vi "1608fsdr_v2.vi"() -> ()   [LabVIEW 2009]
uses:
  Das16.llb/FromEng(trigger).VI
  Das16.llb/ToEng(array).vi
  PD_Filepath.vi
  Global 2.vi
  Global 3.vi
  DAQGlobal.vi
panel:
  in  "Tab Control":enum32{"Setup", "Acquisition"}(tab)
  in  "Type":u32(ring)=12
  in  "LowThreshold\n             (Volts)":sgl min=-10 max=10 format="%.2f"
  in  "HighThreshold \n              (Volts)":sgl=3.0 min=-10 max=10 format="%.2f"
  out "SetTrig ErrMsg":string
  in  "Mode":i32(ring) items=["DEFAULTIO", "SINGLEIO", "DMAIO", "BLOCKIO", "BURSTIO"]
  in  "Extclock":bool
  in  "BoardNum":u32=1
  in  "Count":i32=1000
  in  "Rate":i32=5000
  in  "LowChan":i32
  in  "HighChan":i32=4
  out "Actual Rate":i32=1000
  in  "Range":i32(ring)=1 items=["Not Programmable"=0, "+- 20 V"=27, "+- 10 V"=1, "+- 5 V"=2, "+- 4 V"=28, "+- 2.5 V"=3, "+- 2 V"=29, "+- 1.67 V"=4, "+- 1.25 V"=5, "+- 1 V"=6, "+- .625 V"=7, "+- .5 V"=8, "+- .25 V"=30, "+- .2 V"=31, "+- .1 V"=9, "+- .05 V"=10, "+- .01 V"=11, "+- .005 V"=12, "0 - 10 V"=13, "0 - 5 V"=14, "0 - 4 V"=36, "0 - 2.5 V"=15, "0 - 2 V"=16, "0 - 1.67 V"=17, "0 - 1.25 V"=18, "0 - 1 V"=19, "0 - .5 V"=32, "0 - .25 V"=33, "0 - .2 V"=34, "0 - .1 V"=20, "0 - .02 V"=35, "0 - .01 V"=21, "4 - 20 mA"=22, "2 - 10 mA"=23, "1 - 5 mA"=24, ".5 - 2.5 mA"=25, "0 - 20 mA"=26]
  in  "InterChannel Delay":dbl=-1.0 format="%.2f"
  in  "ExtTrigger":bool
  out "Count/Channel":u32=500
  out "Channel Count":u32=2
  in  "stop 2":bool
  in  "time format string (%c)":string
  in  "width (-)":i16
  in  "precision (6)":i16
  out "Complete data output path":path=path "C:/Docs/LabVIEW Data/Acquisition.lvm" caption="File Name Out"
  out "Statistics filename":string
  out "Saving?":bool
  out "Streaming data":sgl[][](graph)
  out "Instantaneous data":sgl[][](graph)=[[-0.009002686, -0.00869751, -0.008392334, -0.007019043, -0.0015258789, -0.00793457, -0.0073242188, 0.00076293945, -0.00579834, -0.007171631, 0.0022888184, 0.0048828125, 0.0010681152, 0.008087158, 0.0064086914, -0.0025939941, 0.0033569336, 0.0051879883, -0.007019043, -0.007019043, -0.004119873, 0.0061035156, 0.00015258789, -0.0022888184, -0.0047302246, -0.0064086914, -0.0047302246, 0.0074768066, 0.0074768066, 0.004119873, 0.009002686, 0.008544922, 0.0018310547, 0.00579834, 0.006866455, -0.0032043457, -0.009155273, -0.0032043457, -0.0059509277, 0.00015258789, 0.0032043457, -0.0018310547, -0.00091552734, -0.007019043, 0.0035095215, 0.0051879883, -0.004272461, -0.00579834, -0.006713867, 0.004272461, -0.0036621094, 0.00579834, 0.00030517578, -0.0030517578, 0.0073242188, 0.0015258789, 0.00030517578, -0.007019043, 0.008087158, 0.004119873, -0.007019043, -0.0038146973, -0.00579834, 0.0048828125, 0.0064086914, 0.0073242188, -0.0076293945, -0.00793457, -0.0021362305, 0.00579834, 0.0048828125, -0.00793457, -0.0051879883, -0.00091552734, 0.007171631, 0.003967285, 0.007171631, -0.0047302246, -0.007019043, 0.005340576, 0.008392334, 0.0022888184, -0.0045776367, -0.0015258789, -0.008239746, -0.0030517578, 0.004272461, -0.00030517578, 0.007171631, 0.0048828125, -0.0019836426, 0.0010681152, 0.00030517578, 0.0076293945, 0.00030517578, -0.0030517578, 0.008392334, 0.009002686, 0.008239746, -0.006866455, 0.0018310547, -0.0064086914, -0.0032043457, 0.0010681152, -0.00793457, -0.00061035156, 0.0012207031, 0.0073242188, -0.0061035156, -0.0018310547, 0.0076293945, 0.0024414062, 0.007019043, -0.0050354004, -0.0059509277, -0.00579834, 0.008850098, 0.0064086914, 0.0, -0.009002686, -0.006713867, 0.007171631, 0.0050354004, 0.00076293945, -0.009307861, -0.0010681152, -0.007171631, -0.0032043457, 0.0048828125, -0.00076293945, 0.0045776367, 0.00793457, 0.0048828125, -0.0033569336, 0.001373291, 0.005493164, -0.0047302246, 0.0, -0.0076293945, -0.0050354004, 0.00045776367, 0.0010681152, 0.0051879883, -0.0061035156, -0.00289917, -0.00015258789, -0.0021362305, -0.0045776367, -0.0062561035, -0.0012207031, -0.00869751, -0.0025939941, 0.0059509277, 0.0032043457, 0.0035095215, 0.00579834, 0.003967285, -0.0045776367, 0.0064086914, 0.008392334, -0.0016784668, -0.007171631, -0.0047302246, 0.005493164, 0.00793457, 0.008087158, -0.005340576, -0.0050354004, -0.0047302246, 0.0038146973, 0.004272461, -0.0064086914, -0.0062561035, -0.0062561035, 0.00793457, -0.0016784668, 0.0074768066, 0.0010681152, -0.0030517578, 0.008392334, -0.0019836426, -0.0047302246, -0.0077819824, 0.004119873, -0.00015258789, -0.008239746, -0.0030517578, -0.007171631, 0.004272461, 0.0061035156, 0.0065612793, -0.0064086914, -0.004119873, -0.006866455, -0.0012207031, 0.00015258789, -0.0016784668, 0.009155273, 0.007019043, -0.0012207031, -0.008239746, -0.00793457, 0.0038146973, 0.0051879883, -0.003967285, 0.007019043, 0.00793457, 0.0019836426, -0.00061035156, 0.0015258789, 0.0074768066, 0.0021362305, 0.0065612793, -0.0045776367, -0.0032043457, 0.0033569336, 0.0022888184, 0.003967285, -0.006713867, -0.005340576, -0.0051879883, 0.0038146973, 0.0019836426, 0.0, -0.00793457, 0.00076293945, -0.0061035156, 0.00289917, 0.0074768066, -0.0038146973, 0.008392334, 0.008087158, 0.004425049, 0.00045776367, 0.0021362305, 0.0048828125, -0.0047302246, 0.00289917, -0.00793457, -0.0012207031, 0.0035095215, -0.00061035156, 0.0021362305, -0.007019043, 0.0010681152, 0.0024414062, -0.0030517578, -0.0061035156, -0.0076293945, 0.005340576, -0.0062561035, -0.0016784668, 0.0048828125, 0.0015258789, 0.0050354004, 0.004272461, 0.0, -0.0059509277, 0.007171631, 0.008544922, -0.0025939941, -0.007019043, -0.0048828125, 0.008239746, 0.006866455, 0.0074768066, -0.00579834, -0.0032043457, -0.008239746, 0.001373291, 0.0032043457, -0.0062561035, -0.006713867, -0.0048828125, 0.007019043, -0.004272461, 0.0038146973, 0.005340576, -0.00015258789, 0.008239746, 0.0, -0.00015258789, -0.0064086914, 0.006866455, 0.0051879883, -0.0062561035, -0.00869751, -0.00579834, 0.0048828125, 0.0062561035, 0.0076293945, -0.0062561035, -0.0032043457, -0.0062561035, 0.003967285, 0.0074768066, -0.0061035156, -0.004119873, -0.004119873, 0.008392334, -0.004119873, 0.0019836426, 0.003967285, -0.0030517578, 0.006866455, -0.0025939941, 0.007171631, 0.0032043457, -0.0015258789, 0.00579834, -0.0050354004, -0.005645752, -0.0050354004, 0.009307861, 0.008392334, 0.005493164, -0.0061035156, -0.0062561035, -0.006713867, 0.0032043457, 0.0048828125, -0.008087158, -0.0045776367, -0.0025939941, 0.006866455, -0.0033569336, 0.0048828125, 0.0022888184, -0.0038146973, 0.008392334, -0.0045776367, -0.005645752, -0.0045776367, 0.0045776367, 0.00579834, -0.00869751, -0.0076293945, -0.0033569336, 0.006866455, 0.0045776367, -0.00076293945, -0.0048828125, -0.00793457, -0.00015258789, 0.007019043, 0.00579834, -0.00091552734, -0.005645752, -0.0030517578, 0.0064086914, 0.00091552734, 0.006866455, -0.0019836426, -0.00793457, 0.0048828125, -0.0076293945, -0.009002686, -0.007019043, 0.0076293945, 0.006866455, -0.0033569336, -0.0051879883, -0.00076293945, 0.0010681152, -0.00091552734, -0.004272461, 0.00289917, -0.0045776367, 0.005340576, 0.00091552734, -0.00030517578, 0.0061035156, 0.0074768066, 0.0059509277, -0.0022888184, 0.0050354004, 0.0021362305, -0.007019043, -0.0045776367, -0.00579834, 0.0033569336, 0.0024414062, 0.0073242188, -0.0050354004, -0.008392334, 0.0010681152, 0.005493164, 0.0045776367, -0.0051879883, -0.008239746, -0.007171631, 0.008850098, 0.0035095215, 0.0062561035, -0.0045776367, -0.005340576, 0.009002686, 0.004272461, 0.0019836426, -0.0061035156, 0.001373291, -0.00579834, -0.005645752, 0.00030517578, 0.0032043457, 0.0051879883, 0.007019043, 0.006866455, -0.0051879883, -0.0038146973, 0.00793457, 0.0019836426, -0.00076293945, -0.0015258789, -0.00030517578, 0.0010681152, -0.0010681152, 0.0062561035, -0.0025939941, -0.003967285, -0.0048828125, 0.0018310547, -0.0045776367, -0.006713867, 0.0, -0.0062561035, -0.0076293945, 0.0033569336, 0.0062561035, 0.00091552734, 0.004425049, 0.0045776367, -0.0021362305, 0.0022888184, 0.0050354004, 0.0033569336, -0.00793457, -0.005340576, 0.0021362305, 0.0062561035, 0.007019043, -0.0064086914, 0.0021362305, -0.006713867, 0.00015258789, 0.0045776367, -0.005645752, -0.0019836426, -0.0022888184, 0.008850098, -0.0064086914, -0.0016784668, 0.0051879883, 0.00045776367, 0.0062561035, -0.0050354004, -0.0047302246, -0.009307861, 0.008392334, 0.007019043, -0.0019836426, -0.007171631, -0.0038146973, 0.009307861, 0.008850098, 0.0051879883, -0.00793457, -0.00579834, -0.008392334, 0.0010681152, 0.0035095215, -0.00793457, -0.0015258789, 0.0012207031, 0.0074768066, -0.0030517578, 0.0035095215, 0.0045776367, -0.002746582, 0.006866455, -0.0051879883, -0.0073242188, -0.0038146973, 0.0050354004, 0.0030517578, -0.00793457, -0.004119873, -0.0010681152, 0.004119873, -0.00061035156, -0.003967285, -0.00076293945, -0.0059509277, 0.001373291, 0.0064086914, 0.004272461, 0.004119873, 0.009307861, 0.007171631, -0.0047302246], [0.034332275, 0.028381348, 0.025024414, 0.02166748, 0.030212402, 0.032348633, 0.033569336, 0.03692627, 0.036010742, 0.036315918, 0.039215088, 0.04058838, 0.04257202, 0.05050659, 0.050354004, 0.043182373, 0.041656494, 0.03555298, 0.028839111, 0.023651123, 0.024414062, 0.034332275, 0.03555298, 0.03616333, 0.035858154, 0.03616333, 0.03692627, 0.04119873, 0.04196167, 0.04547119, 0.05142212, 0.0491333, 0.04333496, 0.040283203, 0.0340271, 0.0289917, 0.022125244, 0.026397705, 0.032043457, 0.034942627, 0.037384033, 0.03692627, 0.038146973, 0.036621094, 0.040130615, 0.043182373, 0.045928955, 0.048217773, 0.04348755, 0.042419434, 0.036010742, 0.032806396, 0.02822876, 0.023345947, 0.032043457, 0.035247803, 0.036315918, 0.034942627, 0.03982544, 0.03982544, 0.037078857, 0.03845215, 0.041046143, 0.049438477, 0.049743652, 0.04562378, 0.038604736, 0.032196045, 0.029754639, 0.02746582, 0.027160645, 0.03036499, 0.033111572, 0.035858154, 0.0390625, 0.03845215, 0.04058838, 0.038146973, 0.037841797, 0.04623413, 0.051574707, 0.047912598, 0.04135132, 0.0390625, 0.030212402, 0.028839111, 0.025482178, 0.027008057, 0.035858154, 0.037078857, 0.036315918, 0.037384033, 0.037841797, 0.041046143, 0.040130615, 0.041046143, 0.048980713, 0.05218506, 0.047912598, 0.040130615, 0.03829956, 0.029449463, 0.027008057, 0.024108887, 0.027923584, 0.034179688, 0.03616333, 0.0390625, 0.03555298, 0.037994385, 0.041046143, 0.04058838, 0.044555664, 0.047302246, 0.047302246, 0.042419434, 0.04333496, 0.036315918, 0.03112793, 0.023956299, 0.023345947, 0.034484863, 0.036621094, 0.037078857, 0.034484863, 0.037841797, 0.03692627, 0.037994385, 0.041046143, 0.044555664, 0.05065918, 0.04928589, 0.044555664, 0.038146973, 0.032958984, 0.03173828, 0.023651123, 0.02746582, 0.03173828, 0.0340271, 0.036621094, 0.037994385, 0.040283203, 0.037384033, 0.038604736, 0.041503906, 0.04623413, 0.048980713, 0.0440979, 0.04119873, 0.03540039, 0.030212402, 0.030212402, 0.025024414, 0.030212402, 0.036315918, 0.037384033, 0.036010742, 0.039367676, 0.040893555, 0.038604736, 0.037994385, 0.041503906, 0.049743652, 0.05050659, 0.046539307, 0.039978027, 0.033569336, 0.029449463, 0.027770996, 0.026245117, 0.030822754, 0.03326416, 0.034484863, 0.039215088, 0.037231445, 0.041046143, 0.039978027, 0.039367676, 0.04699707, 0.04928589, 0.046539307, 0.041046143, 0.040893555, 0.03326416, 0.028076172, 0.023651123, 0.025177002, 0.034484863, 0.037078857, 0.038604736, 0.035858154, 0.037384033, 0.03692627, 0.038909912, 0.04135132, 0.04623413, 0.052642822, 0.048065186, 0.041503906, 0.03616333, 0.029144287, 0.029449463, 0.02532959, 0.028076172, 0.036621094, 0.038146973, 0.038146973, 0.037231445, 0.038909912, 0.04135132, 0.04058838, 0.044555664, 0.047302246, 0.048065186, 0.045166016, 0.042114258, 0.036468506, 0.029754639, 0.025482178, 0.023345947, 0.033569336, 0.036010742, 0.03692627, 0.035095215, 0.03829956, 0.037384033, 0.03982544, 0.042114258, 0.043029785, 0.051574707, 0.049743652, 0.044708252, 0.03982544, 0.03326416, 0.032196045, 0.023651123, 0.02822876, 0.03173828, 0.035095215, 0.037841797, 0.037841797, 0.039215088, 0.037231445, 0.039520264, 0.04196167, 0.04562378, 0.04852295, 0.0440979, 0.04348755, 0.036468506, 0.03112793, 0.03036499, 0.025024414, 0.03036499, 0.03616333, 0.036468506, 0.035858154, 0.039520264, 0.04135132, 0.038604736, 0.038146973, 0.041656494, 0.05065918, 0.05065918, 0.04699707, 0.040283203, 0.035247803, 0.0289917, 0.027008057, 0.025939941, 0.030517578, 0.033111572, 0.035247803, 0.039367676, 0.036621094, 0.040130615, 0.04135132, 0.04043579, 0.046539307, 0.050048828, 0.048217773, 0.04196167, 0.042114258, 0.03540039, 0.029449463, 0.02243042, 0.025482178, 0.034942627, 0.037384033, 0.0390625, 0.035858154, 0.037841797, 0.037384033, 0.04043579, 0.043182373, 0.044555664, 0.048980713, 0.045166016, 0.044555664, 0.037231445, 0.032196045, 0.030517578, 0.023956299, 0.030822754, 0.034332275, 0.03829956, 0.03845215, 0.037384033, 0.04058838, 0.038146973, 0.03845215, 0.041656494, 0.051116943, 0.051727295, 0.046691895, 0.040130615, 0.034484863, 0.029296875, 0.027770996, 0.02609253, 0.029907227, 0.03387451, 0.035858154, 0.039520264, 0.036621094, 0.04043579, 0.04043579, 0.039367676, 0.046691895, 0.048675537, 0.046691895, 0.042419434, 0.04196167, 0.03555298, 0.028381348, 0.023040771, 0.026245117, 0.03555298, 0.03753662, 0.037231445, 0.036010742, 0.036315918, 0.038909912, 0.04196167, 0.043029785, 0.04623413, 0.048675537, 0.04562378, 0.044708252, 0.038604736, 0.03387451, 0.029296875, 0.02243042, 0.030059814, 0.032958984, 0.034179688, 0.03540039, 0.040130615, 0.040893555, 0.03845215, 0.03845215, 0.043182373, 0.048675537, 0.049743652, 0.04425049, 0.042266846, 0.035095215, 0.032958984, 0.02822876, 0.025024414, 0.033416748, 0.03753662, 0.038604736, 0.037231445, 0.03982544, 0.040130615, 0.037841797, 0.038909912, 0.042114258, 0.050354004, 0.048980713, 0.04623413, 0.039215088, 0.03189087, 0.03112793, 0.026855469, 0.028839111, 0.03250122, 0.033569336, 0.035095215, 0.040130615, 0.039367676, 0.04135132, 0.0390625, 0.03982544, 0.04852295, 0.051727295, 0.047912598, 0.04135132, 0.03982544, 0.03112793, 0.028076172, 0.024719238, 0.029296875, 0.03616333, 0.038146973, 0.039367676, 0.036468506, 0.037841797, 0.041503906, 0.04119873, 0.04333496, 0.047454834, 0.049591064, 0.04547119, 0.04196167, 0.0390625, 0.031280518, 0.027160645, 0.023040771, 0.032806396, 0.034484863, 0.035247803, 0.037384033, 0.03692627, 0.037384033, 0.040283203, 0.04196167, 0.04348755, 0.051116943, 0.050354004, 0.043945312, 0.04135132, 0.035858154, 0.032806396, 0.023803711, 0.025787354, 0.034179688, 0.03753662, 0.039215088, 0.036315918, 0.039520264, 0.037841797, 0.03982544, 0.042114258, 0.044403076, 0.04928589, 0.046539307, 0.04547119, 0.03753662, 0.032043457, 0.03173828, 0.02532959, 0.029754639, 0.033569336, 0.035247803, 0.035095215, 0.04043579, 0.04119873, 0.0390625, 0.03829956, 0.042114258, 0.05050659, 0.052490234, 0.047454834, 0.040130615, 0.03616333, 0.029449463, 0.02822876, 0.025787354, 0.029449463, 0.034942627, 0.03692627, 0.039978027, 0.037384033, 0.04043579, 0.04135132, 0.040130615, 0.04547119, 0.048217773, 0.04699707, 0.043182373, 0.04257202, 0.035858154, 0.029144287, 0.024414062, 0.02670288, 0.035247803, 0.03616333, 0.036621094, 0.037384033, 0.037078857, 0.03982544, 0.042114258, 0.042114258, 0.04699707, 0.05279541, 0.049591064, 0.042266846]]
  in  "Filepath":string="c:\\Docs\\Labview data\\tests\\"
  in  "Filter under test":string="filter"
  out "Present wavelength (nm)":dbl
  out "date/time string":string
  out "F-format string":string
  out "Shutter Status":bool caption="OK Button"
  out "Average Ch0 and 1":dbl[][](array[numeric])=[[-1.03759765625e-05, 0.0377886962890625]]
  out "Max range Ch0 and 1":dbl[][](array[numeric])=[[0.01861572265625, 0.0311279296875]]
  out "Statistics output path":path=path "C:/Docs/LabVIEW Data/Acquisition.lvm" caption="File Name Out"
  out "Complete data filename":string
  out "ErrMsg":string="No error has occurred"
  out "CurCount":i32=1000
  out "DataArray":u16[](array[numeric])=[32709, 32993, 32711, 32954, 32713, 32932, 32722, 32910, 32758, 32966, 32716, 32980, 32720, 32988, 32773, 33010, 32730, 33004, 32721, 33006, 32783, 33025, 32800, 33034, 32775, 33047, 32821, 33099, 32810, 33098, 32751, 33051, 32790, 33041, 32802, 33001, 32722, 32957, 32722, 32923, 32741, 32928, 32808, 32993, 32769, 33001, 32753, 33005, 32737, 33003, 32726, 33005, 32737, 33010, 32817, 33038, 32817, 33043, 32795, 33066, 32827, 33105, 32824, 33090, 32780, 33052, 32806, 33032, 32813, 32991, 32747, 32958, 32708, 32913, 32747, 32941, 32729, 32978, 32769, 32997, 32789, 33013, 32756, 33010, 32762, 33018, 32722, 33008, 32791, 33031, 32802, 33051, 32740, 33069, 32730, 33084, 32724, 33053, 32796, 33046, 32744, 33004, 32806, 32983, 32770, 32953, 32748, 32921, 32816, 32978, 32778, 32999, 32770, 33006, 32722, 32997, 32821, 33029, 32795, 33029, 32722, 33011, 32743, 33020, 32730, 33037, 32800, 33092, 32810, 33094, 32816, 33067, 32718, 33021, 32716, 32979, 32754, 32963, 32806, 32948, 32800, 32946, 32716, 32967, 32734, 32985, 32762, 33003, 32815, 33024, 32794, 33020, 32815, 33034, 32737, 33018, 32722, 33016, 32803, 33071, 32823, 33106, 32783, 33082, 32738, 33039, 32758, 33024, 32714, 32966, 32748, 32957, 32796, 32935, 32766, 32945, 32815, 33003, 32800, 33011, 32755, 33006, 32775, 33013, 32770, 33016, 32818, 33037, 32770, 33031, 32748, 33037, 32823, 33089, 32827, 33110, 32822, 33082, 32723, 33031, 32780, 33019, 32726, 32961, 32747, 32945, 32775, 32926, 32716, 32951, 32764, 32992, 32776, 33005, 32816, 33024, 32728, 33001, 32756, 33017, 32818, 33037, 32784, 33034, 32814, 33060, 32735, 33078, 32729, 33078, 32730, 33046, 32826, 33052, 32810, 33006, 32768, 32972, 32709, 32925, 32724, 32921, 32815, 32994, 32801, 33008, 32773, 33011, 32707, 32994, 32761, 33016, 32721, 33010, 32747, 33017, 32800, 33037, 32763, 33060, 32798, 33100, 32820, 33091, 32800, 33060, 32746, 33018, 32777, 32984, 32804, 32976, 32737, 32923, 32768, 32948, 32718, 32976, 32735, 32991, 32771, 33008, 32775, 33017, 32802, 33032, 32728, 33013, 32749, 33021, 32767, 33040, 32754, 33071, 32738, 33089, 32727, 33057, 32760, 33038, 32711, 33000, 32751, 32966, 32807, 32966, 32789, 32932, 32791, 32966, 32806, 33006, 32794, 33013, 32738, 33004, 32810, 33026, 32823, 33036, 32757, 33021, 32721, 33017, 32737, 33040, 32804, 33094, 32820, 33099, 32821, 33073, 32733, 33030, 32735, 32988, 32737, 32961, 32793, 32950, 32796, 32940, 32726, 32970, 32727, 32986, 32727, 32994, 32820, 33025, 32757, 33012, 32817, 33037, 32775, 33030, 32748, 33026, 32823, 33076, 32755, 33091, 32737, 33073, 32717, 33037, 32795, 33036, 32767, 32986, 32714, 32952, 32748, 32923, 32721, 32933, 32796, 32994, 32808, 33011, 32811, 33021, 32726, 33003, 32741, 33013, 32723, 33010, 32760, 33023, 32769, 33039, 32757, 33071, 32828, 33113, 32814, 33083, 32760, 33040, 32714, 33005, 32716, 32959, 32793, 32961, 32802, 32934, 32742, 32952, 32814, 33008, 32820, 33018, 32781, 33018, 32764, 33012, 32778, 33023, 32817, 33039, 32782, 33034, 32811, 33060, 32738, 33078, 32747, 33083, 32790, 33064, 32783, 33044, 32794, 33007, 32724, 32963, 32733, 32935, 32734, 32921, 32793, 32988, 32781, 33004, 32768, 33010, 32716, 32998, 32773, 33019, 32728, 33013, 32787, 33029, 32817, 33044, 32743, 33050, 32823, 33106, 32821, 33094, 32797, 33061, 32771, 33029, 32782, 32986, 32800, 32979, 32737, 32923, 32787, 32953, 32716, 32976, 32760, 32998, 32791, 33016, 32764, 33016, 32782, 33025, 32722, 33012, 32775, 33027, 32784, 33043, 32748, 33067, 32728, 33086, 32718, 33057, 32803, 33053, 32727, 33007, 32757, 32972, 32800, 32967, 32778, 32932, 32801, 32967, 32796, 33005, 32768, 33007, 32729, 33003, 32815, 33027, 32824, 33039, 32751, 33021, 32722, 33018, 32736, 33041, 32822, 33100, 32813, 33100, 32817, 33076, 32730, 33032, 32747, 32999, 32714, 32958, 32777, 32945, 32789, 32938, 32727, 32968, 32724, 32985, 32736, 32999, 32814, 33026, 32740, 33008, 32793, 33031, 32803, 33039, 32767, 33033, 32822, 33073, 32768, 33096, 32767, 33084, 32726, 33043, 32813, 33044, 32802, 33000, 32727, 32961, 32711, 32915, 32730, 32935, 32800, 32997, 32809, 33013, 32818, 33024, 32727, 33003, 32747, 33016, 32727, 33013, 32794, 33033, 32817, 33051, 32728, 33060, 32741, 33089, 32741, 33064, 32823, 33060, 32741, 33012, 32781, 32979, 32794, 32968, 32748, 32925, 32813, 32970, 32751, 32993, 32815, 33019, 32789, 33020, 32758, 33013, 32806, 33034, 32735, 33018, 32731, 33020, 32735, 33041, 32829, 33103, 32823, 33107, 32804, 33074, 32728, 33031, 32727, 32994, 32724, 32960, 32789, 32950, 32800, 32939, 32715, 32964, 32738, 32990, 32751, 33003, 32813, 33027, 32746, 33008, 32800, 33033, 32783, 33033, 32743, 33026, 32823, 33074, 32738, 33087, 32731, 33074, 32738, 33046, 32798, 33043, 32806, 33001, 32711, 32954, 32718, 32919, 32746, 32940, 32813, 33001, 32798, 33014, 32763, 33012, 32736, 33004, 32716, 33006, 32767, 33023, 32814, 33043, 32806, 33050, 32762, 33071, 32731, 33087, 32748, 33067, 32810, 33061, 32774, 33021, 32813, 32990, 32755, 32960, 32716, 32915, 32800, 32965, 32718, 32984, 32709, 32992, 32722, 33000, 32818, 33031, 32813, 33036, 32746, 33020, 32734, 33020, 32763, 33051, 32775, 33087, 32762, 33094, 32740, 33058, 32787, 33045, 32738, 32998, 32803, 32984, 32774, 32953, 32766, 32932, 32808, 32987, 32817, 33014, 32807, 33021, 32753, 33012, 32801, 33029, 32782, 33031, 32722, 33016, 32738, 33023, 32730, 33044, 32790, 33098, 32784, 33089, 32816, 33071, 32735, 33025, 32713, 32977, 32775, 32972, 32804, 32944, 32798, 32957, 32734, 32981, 32714, 32988, 32721, 32998, 32826, 33031, 32791, 33026, 32809, 33039, 32738, 33024, 32733, 33029, 32827, 33086, 32796, 33107, 32781, 33082, 32728, 33039, 32777, 33029, 32730, 32972, 32731, 32952, 32770, 32930, 32789, 32960, 32802, 33005, 32814, 33018, 32813, 33026, 32734, 33007, 32743, 33016, 32820, 33040, 32781, 33038, 32763, 33052, 32758, 33079, 32766, 33093, 32775, 33066, 32761, 33043, 32809, 33024, 32751, 32973, 32742, 32946, 32736, 32919, 32780, 32983, 32738, 32994, 32724, 32999, 32768, 33013, 32727, 33010, 32718, 33013, 32790, 33032, 32809, 33043, 32774, 33053, 32797, 33103, 32798, 33098, 32754, 33056, 32783, 33039, 32801, 33003, 32790, 32983, 32716, 32924, 32733, 32937, 32782, 32992, 32809, 33014, 32814, 33025, 32726, 33006, 32782, 33027, 32724, 33016, 32769, 33029, 32798, 33044, 32731, 33059, 32755, 33091, 32753, 33073, 32826, 33066, 32726, 33014, 32757, 32978, 32802, 32976, 32771, 32934, 32809, 32963, 32735, 32988, 32737, 32999, 32707, 32998, 32823, 33033, 32814, 33038, 32755, 33024, 32721, 33019, 32743, 33044, 32829, 33099, 32826, 33112, 32802, 33079, 32716, 33031, 32730, 33005, 32713, 32961, 32775, 32953, 32791, 32937, 32716, 32961, 32758, 32997, 32776, 33010, 32817, 33030, 32748, 33013, 32791, 33033, 32798, 33039, 32750, 33031, 32813, 33066, 32734, 33084, 32720, 33076, 32743, 33051, 32801, 33047, 32788, 33003, 32716, 32959, 32741, 32928, 32761, 32943, 32795, 32999, 32764, 33005, 32742, 33008, 32763, 33013, 32729, 33011, 32777, 33029, 32810, 33044, 32796, 33044, 32795, 33076, 32829, 33114, 32815, 33093, 32737, 33045]
  in  "Abort Acquisition":bool
  # "SetTrig.VI input parameters:"
  # "Options parameters (input to OptAIn.VI).\nDefault used for other option parameters."
  # "AInScBg.VI input parameters:"
  # "StopBg.VI output:"
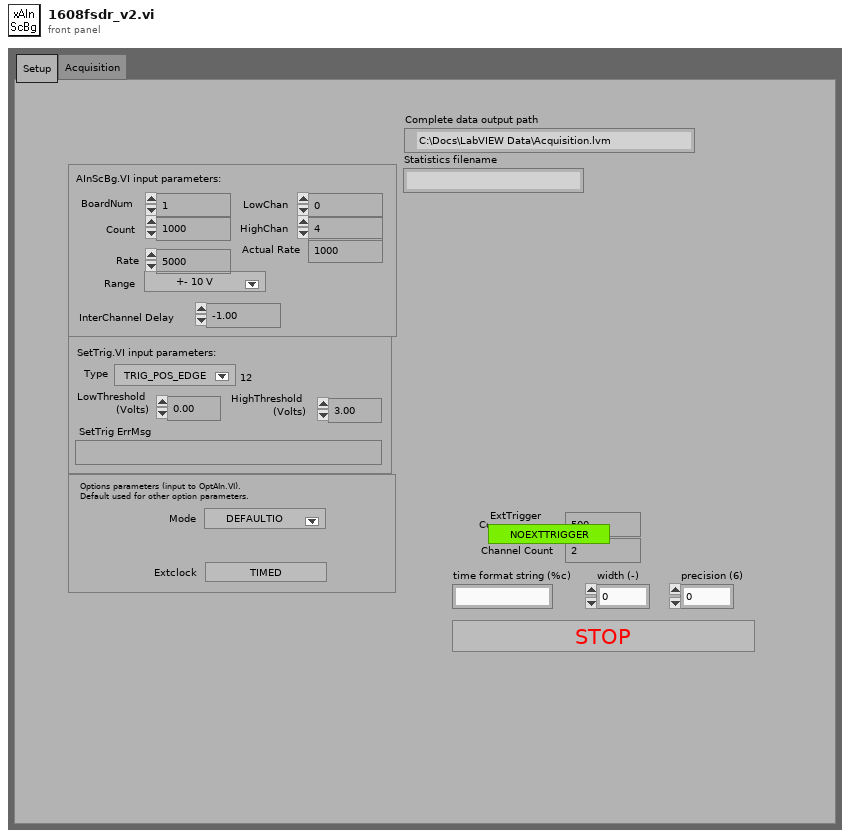
[diagram p1: front panel]
types:
  T1 = cluster{"IntnlBoardNum":i32, "Data":i16[], "Size":i32, "IntnlStatus":i32, "IntnlErrCode":i32, "Alias16":u32, "Reserved":i32}
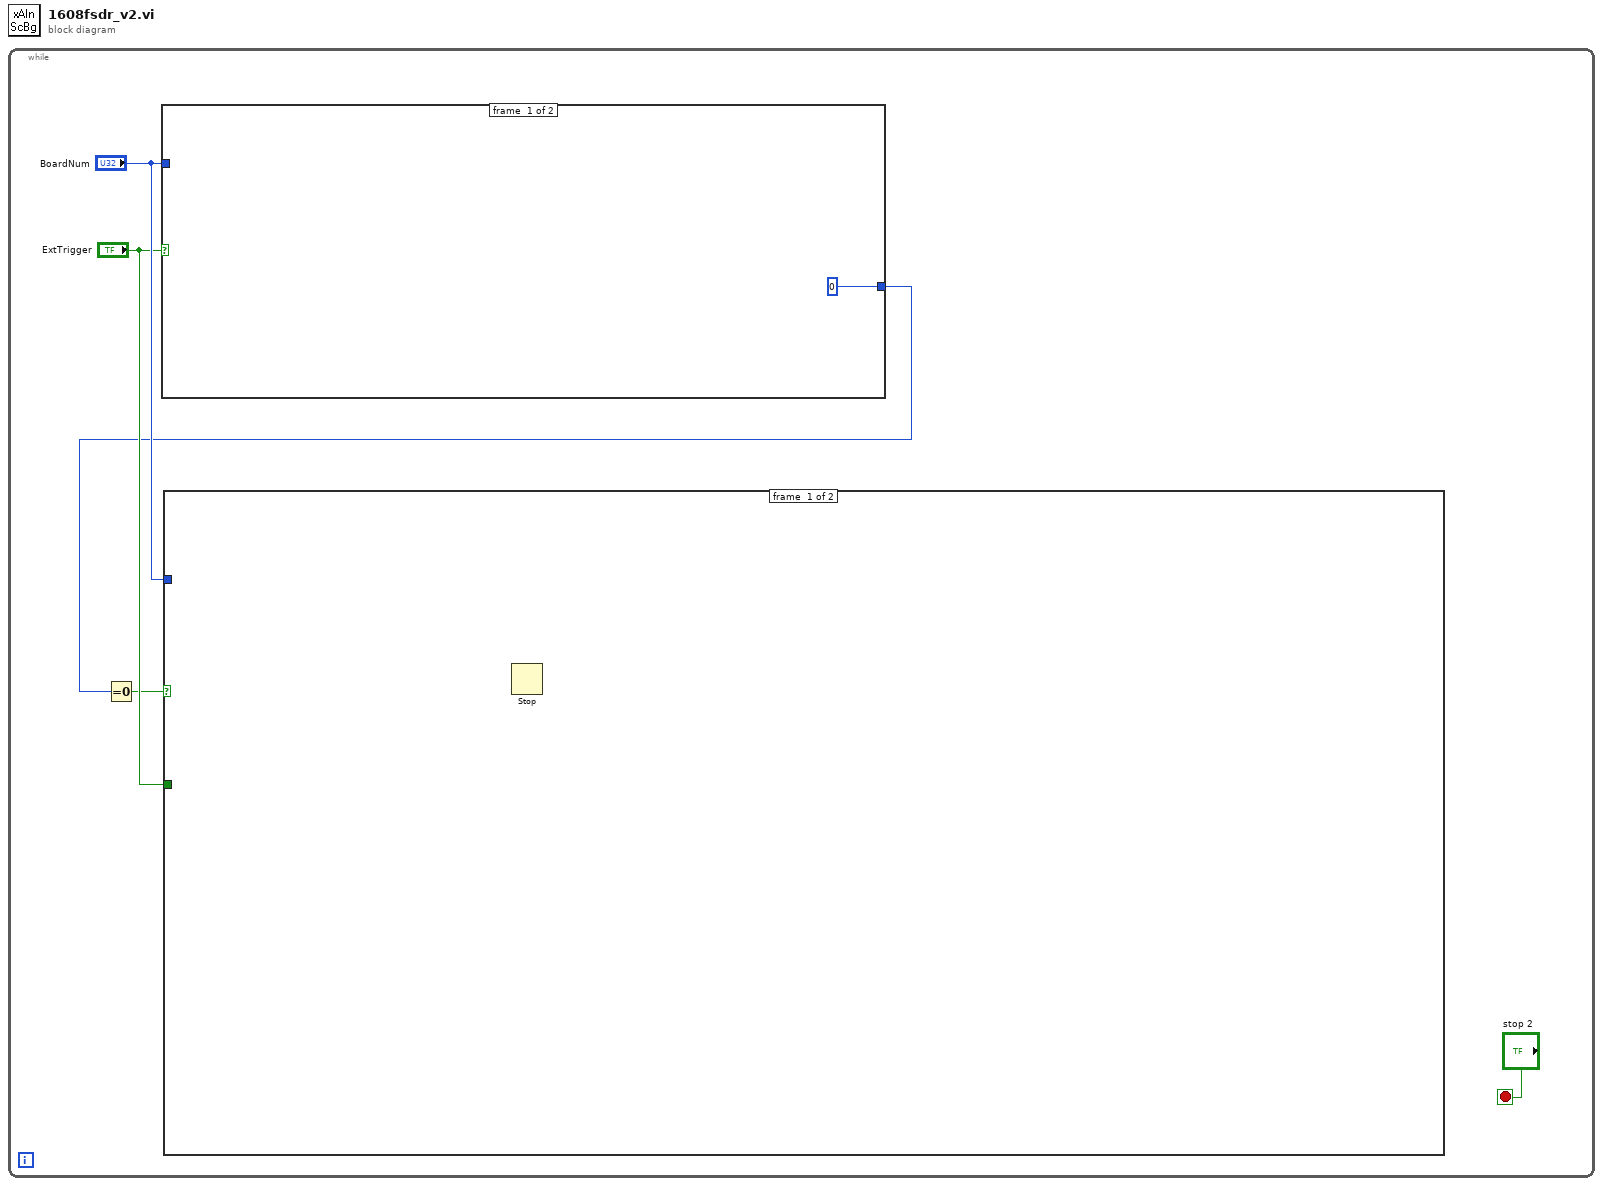
[diagram p0: block diagram]
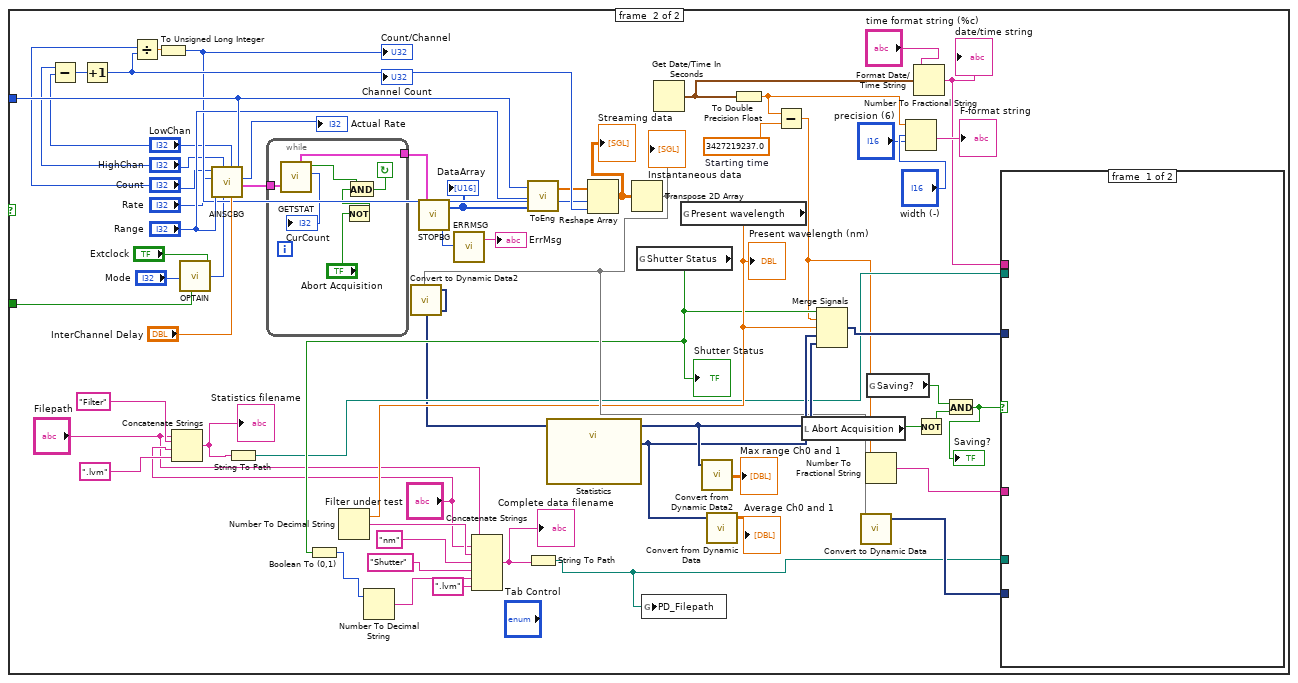
[diagram p2: hidden frame]
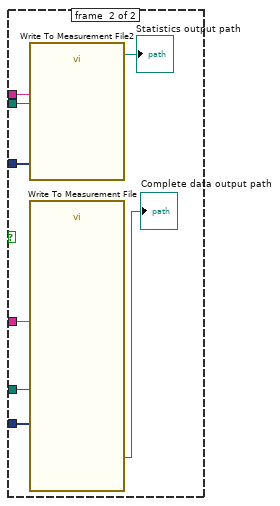
[diagram p3: hidden frame]
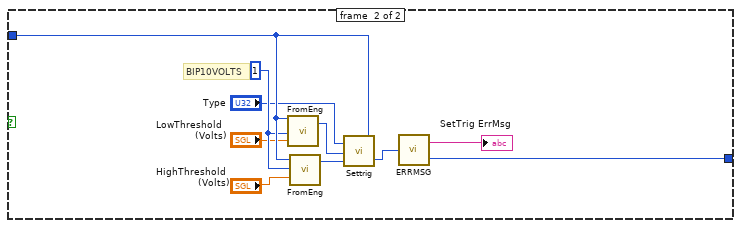
[diagram p4: hidden frame]
diagram:
  n1 = while {
    stop <- "stop 2" stop-if-true
    n2 = case shown="True" "ExtTrigger" {
      tunnel: "BoardNum" -> [_ w92]
      tunnel: [0 w83] -> w3
      frame #0 {
      }
      frame #1 {
        w91 = 1
        # "BIP10VOLTS"
        n3 = call-poly "FromEng.VI"("Eng Units"="LowThreshold\n             (Volts)", "Range"=w91, "BoardNum (0)"=w92) -> ("Threshold Data"=w86:u16)  [unwired: 1 out]
        n4 = call-poly "FromEng.VI"("Eng Units"="HighThreshold \n              (Volts)", "Range"=w91, "BoardNum (0)"=w92) -> ("Threshold Data"=w85:u16)  [unwired: 1 out]
        n5 = call "Settrig.VI"("BoardNum(0)"=w92, "HighThreshold (Counts)"=w85, "LowThreshold (Counts)"=w86, "Type"="Type") -> ("ErrCode"=w84:i32)
        n6 = call "ERRMSG.VI"("ErrCode"=w84) -> ("ErrMsg"=→"SetTrig ErrMsg":string, "ErrCode (Out)"=w83:i32)
      }
    }
    n7 = Equal To 0?(x=w3) -> (x = 0?=w2:bool)
    n8 = case shown="True" w2 {
      tunnel: "BoardNum" -> [_ w66]
      tunnel: "ExtTrigger" -> [_ w65]
      frame #0 {
        n9 = Stop() -> ()  [unwired: 1 in]
      }
      frame #1 {
        w38 = 3427219237.0  # Starting time
        n10 = Subtract(x="HighChan", y="LowChan") -> (x-y=w58:i32)
        n11 = Increment(x=w58) -> (x+1=w63:i32)
        "Channel Count" <- w63
        n12 = Divide(x="Count", y=w63) -> (x/y=w59:dbl)
        n13 = To Unsigned Long Integer(number=w59) -> (unsigned 32bit integer=w60:u32)
        "Count/Channel" <- w60
        n14 = Concatenate Strings("Filepath", "Filter" ("string"), "Filter under test", ".lvm" ("string")) -> (w20:string)
        "Statistics filename" <- w20
        n15 = call "OPTAIN.VI"("Mode"="Mode", "ExtTrigger(false)"=w65, "Extclock(false)"="Extclock") -> ("AInScanOptions"=w49:u32)  [unwired: 6 in]
        n16 = call "AINSCBG.VI"("BoardNum"=w66, "InterChannel Delay"="InterChannel Delay", "LowChan"="LowChan", "Options"=w49, "HighChan"="HighChan", "Range"="Range", "Rate"="Rate", "Count"="Count") -> ("Context"=w48:T1, "Rate"=→"Actual Rate":i32)  [unwired: 1 in, 1 out]
        n17 = String To Path(string=w20) -> (path=w18:path)
        n18 = while {
          tunnel: [w81] -> w57
          tunnel: w48 -> [w75]
          stop <- w78 continue-if-true
          n19 = call "GETSTAT.VI"("Context"=w75) -> ("Context"=w81:T1, "Running"=w77:bool, "CurCount"=→"CurCount":i32)  [unwired: 1 in, 3 out]
          n20 = Not(x="Abort Acquisition") -> (.not. x?=w76:bool)
          n21 = And(x=w77, y=w76) -> (x .and. y?=w78:bool)
        }
        n22 = call "STOPBG.VI"("Context"=w57) -> ("ErrorCode"=w46:i32, "Data"=w54:u16[])  [unwired: 1 in]
        "DataArray" <- w54
        n23 = call "ERRMSG.VI"("ErrCode"=w46) -> ("ErrMsg"=→"ErrMsg":string)  [unwired: 1 out]
        n24 = call-poly "ToEng.VI"("AD Data"=w54, "Range"="Range", "BoardNum"=w66) -> ("Eng Units"=w62:sgl[])  [unwired: 1 out]
        n25 = Reshape Array(w62, w60, w63) -> (w15:sgl[][])
        "Streaming data" <- w15
        n26 = Transpose 2D Array(2D array=w15) -> (transposed array=w32:sgl[][])
        "Instantaneous data" <- w32
        n27 = call "Convert to Dynamic Data2"("2D Array"=w32) -> ("Dynamic Data Type"=w16:dynamicdata)  [unwired: 3 in]
        n28 = call "Statistics"("Signals"=w16) -> ("Arithmetic Mean"=w33:dynamicdata, "Range"=w34:dynamicdata)  [unwired: 23 in, 2 out]
        n29 = global read "Global 3.vi" "Shutter Status"() -> (w25:bool)
        "Shutter Status" <- w25
        n30 = Boolean To (0,1)(Boolean=w25) -> (0, 1=w24:i16)
        n31 = Number To Decimal String(number=w24) -> (decimal integer string=w23:string)  [unwired: 1 in]
        n32 = Get Date/Time In Seconds() -> (seconds since 1Jan1904=w41:timestamp)
        n33 = global read "Global 2.vi" "Present wavelength"() -> (w27:dbl)
        "Present wavelength (nm)" <- w27
        n34 = Number To Decimal String(number=w27) -> (decimal integer string=w28:string)  [unwired: 1 in]
        n35 = Concatenate Strings("Filepath", "Filter under test", w28, "nm" ("string"), "Shutter" ("string"), w23, ".lvm" ("string")) -> (w29:string)
        "Complete data filename" <- w29
        n36 = String To Path(string=w29) -> (path=w6:path)
        n37 = global write "PD_Filepath.vi" "PD_Filepath"(w6) -> ()
        n38 = call "Convert from Dynamic Data2"("Dynamic Data Type"=w34) -> ("Array"=→"Max range Ch0 and 1":dbl[][])  [unwired: 3 in]
        n39 = call "Convert from Dynamic Data"("Dynamic Data Type"=w33) -> ("Array"=→"Average Ch0 and 1":dbl[][])  [unwired: 3 in]
        n40 = To Double Precision Float(number=w41) -> (double precision float=w36:dbl)
        n41 = Subtract(x=w36, y=w38) -> (x-y=w11:dbl)
        n42 = local read "Abort Acquisition"() -> (w9:bool)
        n43 = Merge Signals(w25, w11, w27, w33, w34) -> (w35:dynamicdata)
        n44 = call "Convert to Dynamic Data"("2D Array"=w32) -> ("Dynamic Data Type"=w31:dynamicdata)  [unwired: 3 in]
        n45 = Number To Fractional String(number=w11) -> (F-format string=w12:string)  [unwired: 3 in]
        n46 = global read "DAQGlobal.vi" "Saving?"() -> (w8:bool)
        n47 = Number To Fractional String(number=w36, width (-)="width (-)", precision (6)="precision (6)") -> (F-format string=→"F-format string":string)  [unwired: 1 in]
        n48 = Format Date/Time String(time format string (%c)="time format string (%c)", seconds (now)=w41) -> (date/time string=w13:string)  [unwired: 1 in]
        "date/time string" <- w13
        n49 = Not(x=w9) -> (.not. x?=w10:bool)
        n50 = And(x=w8, y=w10) -> (x .and. y?=w7:bool)
        "Saving?" <- w7
        n51 = case shown="True" w7 {
          tunnel: w35 -> [_ w73]
          tunnel: w31 -> [_ w72]
          tunnel: w6 -> [_ w70]
          tunnel: w18 -> [_ w69]
          tunnel: w13 -> [_ w68]
          tunnel: w12 -> [_ w67]
          frame #0 {
          }
          frame #1 {
            n52 = call "Write To Measurement File2"("Signals"=w73, "File Name"=w69, "Comment"=w68) -> ("File Name Out"=→"Statistics output path":path)  [unwired: 14 in, 2 out]
            n53 = call "Write To Measurement File"("Signals"=w72, "File Name"=w70, "Comment"=w67) -> ("File Name Out"=→"Complete data output path":path)  [unwired: 14 in, 2 out]
          }
        }
      }
    }
  }
